vi "Calculate defocus.vi"(8 "error in (no error)":errorcluster, 11 "Retiga in":refnum<class "Retiga.lvclass">) -> (0 "error out":errorcluster, 1 "fine?":bool, 2 "translation out":dbl[unit], 3 "Retiga out":refnum<class "Retiga.lvclass">)   [LabVIEW 2012, in "Retiga.lvclass"]
uses:
  Retiga.lvclass
  Retiga.lvclass/Retiga.ctl
  <vilib>/vision/NI_Vision_Development_Module.lvlib
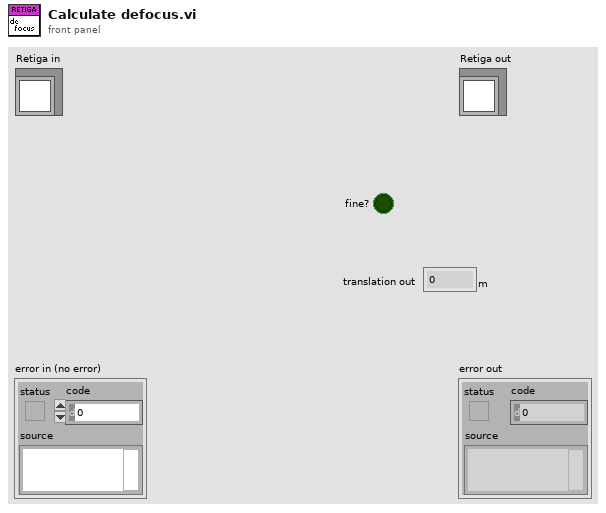
[diagram p1: front panel]
types:
  T1 = typedef "IMAQ Image.ctl" = refnum<image>
  T2 = cluster{"histogram":u32[], "Minimal Value":sgl, "Maximal Value":sgl, "Starting Value":sgl, "Interval Width":sgl, "Mean Value":sgl, "Standard  Variation":sgl, "Area (pixels)":i32}
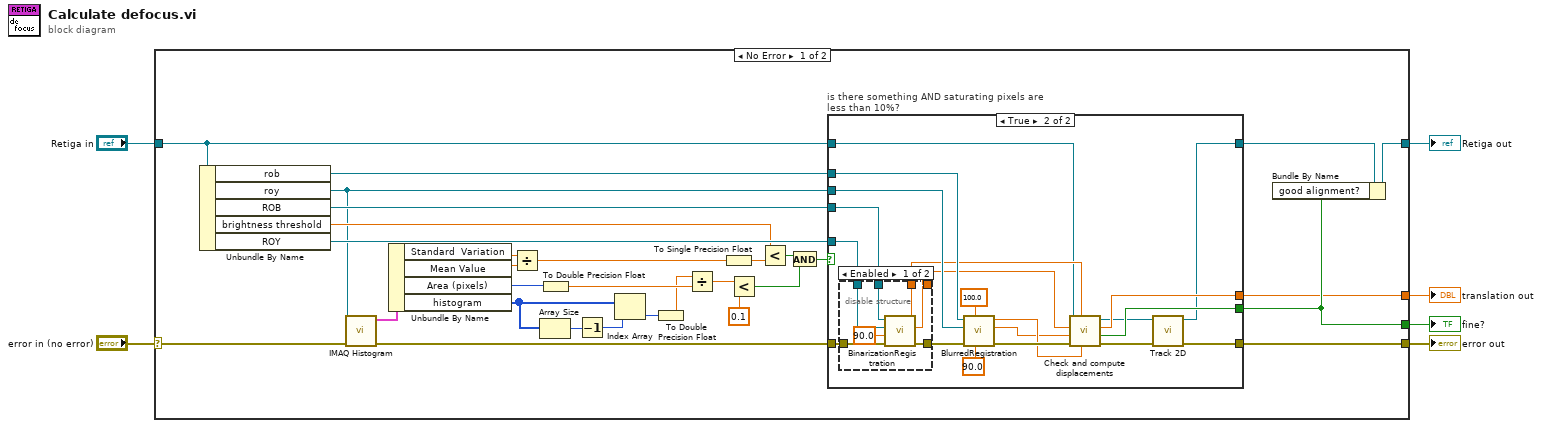
[diagram p0: block diagram]
diagram:
  n1 = case shown="No Error" "error in (no error)" {
    selector: "error in (no error)" -> [w10 w68]
    tunnel: [w9 w68] -> w5
    tunnel: [w11 w67] -> w3
    tunnel: "Retiga in" -> [w12 w67]
    tunnel: [w8 _] -> w2
    tunnel: [w7 _] -> w1
    frame No Error {
      n2 = Unbundle By Name(w12) -> ("rob"=w35:T1, "roy"=w30:T1, "ROB"=w36:T1, "brightness threshold"=w33:sgl, "ROY"=w34:T1)
      n3 = call "IMAQ Histogram"("error in (no error)"=w10, "Image"=w30) -> ("error out"=w31:errorcluster, "Histogram Report"=w29:T2)  [unwired: 8 in]
      n4 = Unbundle By Name(w29) -> ("Standard  Variation"=w28:sgl, "Mean Value"=w27:sgl, "Area (pixels)"=w22:i32, "histogram"=w25:u32[])
      n5 = Divide(x=w28, y=w27) -> (x/y=w26:sgl)
      n6 = Array Size(array=w25) -> (size(s)=w24:i32)
      n7 = To Double Precision Float(number=w22) -> (double precision float=w20:dbl)
      n8 = Decrement(x=w24) -> (x-1=w23:i32)
      n9 = Index Array(array=w25, index=w23) -> (element=w21:u32)
      n10 = To Double Precision Float(number=w21) -> (double precision float=w18:dbl)
      n11 = Divide(x=w18, y=w20) -> (x/y=w19:dbl)
      n12 = To Single Precision Float(number=w26) -> (single precision float=w32:sgl)
      n13 = Less?(x=w19, y=0.1) -> (x < y?=w16:bool)
      n14 = Less?(x=w33, y=w32) -> (x < y?=w15:bool)
      n15 = And(x=w15, y=w16) -> (x .and. y?=w14:bool)
      n16 = case "is there something AND saturating pixels are less than 10%?" shown="True" w14 {
        tunnel: w36 -> [_ w54]
        tunnel: w30 -> [_ w52]
        tunnel: w35 -> [_ w53]
        tunnel: [w38 w39] -> w13
        tunnel: [w37 w41] -> w9
        tunnel: [_ w43] -> w7
        tunnel: [_ w44] -> w8
        tunnel: w12 -> [w38 w45]
        tunnel: w34 -> [_ w51]
        tunnel: w31 -> [w37 w55]
        frame False {
        }
        frame True {
          n17 = disable-structure shown="Enabled" {
            disable-tunnel: [w65 w66] -> w58
            disable-tunnel: w55 -> [w64 w66]
            disable-tunnel: w54 -> [w63 _]
            disable-tunnel: w51 -> [w62 _]
            disable-tunnel: [w60 _] -> w49
            disable-tunnel: [w59 _] -> w46
            frame Enabled {
              n18 = call "BinarizationRegistration.vi"("error in"=w64, "threshold percentage"=90.0, "Roy"=w62, "Rob"=w63) -> ("error out"=w65:errorcluster, "y translation"=w59:dbl, "x translation"=w60:dbl)  [unwired: 4 in, 1 out]
            }
            frame Disabled {
            }
          }
          n19 = call "BlurredRegistration.vi"("small sigma"=sgl 90.0, "large sigma"=sgl 100.0, "error in"=w58, "roy"=w52, "rob"=w53) -> ("error out"=w50:errorcluster, "y displacement"=w47:dbl, "x displacement"=w48:dbl)  [unwired: 3 in, 1 out]
          n20 = call-dynamic "Check and compute displacements.vi"("x pixel displacement 2"=w48, "x pixel displacement 1"=w49, "error in (no error)"=w50, "y pixel displacement 2"=w47, "y pixel displacement 1"=w46, "Retiga in"=w45) -> ("error out"=w42:errorcluster, "fine?"=w44:bool, "translation out"=w43:dbl[unit], "Retiga out"=w40:refnum<class "Retiga.lvclass">)  [unwired: 2 in]
          n21 = call-dynamic "Track 2D.vi"("error in (no error)"=w42, "Retiga in"=w40) -> ("error out"=w41:errorcluster, "Retiga out"=w39:refnum<class "Retiga.lvclass">)  [unwired: 8 in]
        }
      }
      n22 = Bundle By Name(cluster=w13, "good alignment?"=w8) -> (w11:refnum<class "Retiga.lvclass">)
    }
    frame Error {
    }
  }
  "error out" <- w5
  "Retiga out" <- w3
  "fine?" <- w2
  "translation out" <- w1
